vi "Stop IRunable.vi"(8 "error in":errorcluster, 11 "IRunnable Object":refnum<class>) -> (0 "error out":errorcluster, 3 "IRunnable":refnum<class "IRunnable.lvclass">)   [LabVIEW 2024]
uses:
  Source/Interfaces/IRunnable/IRunnable.lvclass
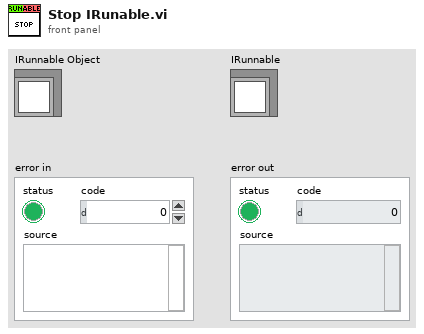
[diagram p1: front panel]
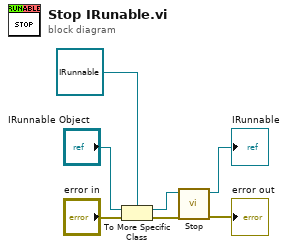
[diagram p0: block diagram]
diagram:
  n1 = To More Specific Class(target class=refnum<class "IRunnable.lvclass"> refnum ("IRunnable.lvclass"), reference="IRunnable Object", error in="error in") -> (specific class reference=w2:refnum<class "IRunnable.lvclass">, error out=w4:errorcluster)
  n2 = call-dynamic "Stop.vi"("error in"=w4, "IRunnable in"=w2) -> ("error out"=→"error out":errorcluster, "IRunnable out"=→"IRunnable":refnum<class "IRunnable.lvclass">)  [unwired: 8 in]
